vi "嵌套条件结构.vi"() -> ()   [LabVIEW 2013]
panel:
  out "output2":dbl
  out "output1":dbl
  out "?":dbl
  out "Array":bool[](array[boolean])
  in  "input":dbl
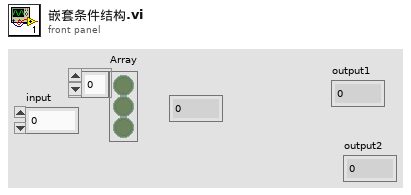
[diagram p1: front panel]
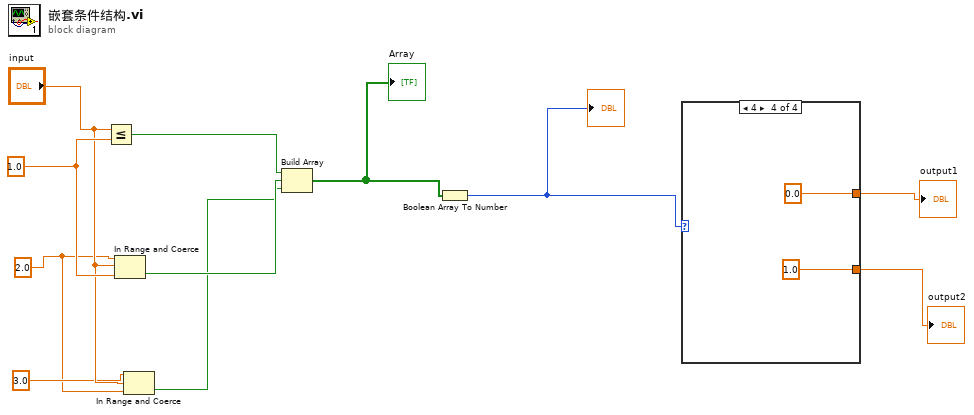
[diagram p0: block diagram]
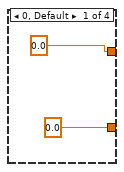
[diagram p2: hidden frame]
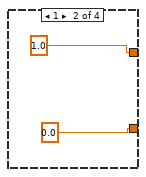
[diagram p3: hidden frame]
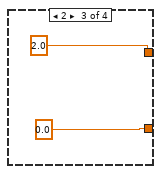
[diagram p4: hidden frame]
diagram:
  w8 = 2.0
  w11 = 1.0
  n1 = Less Or Equal?(x="input", y=w11) -> (x <= y?=w7:bool)
  n2 = In Range and Coerce(upper limit=w8, x="input", lower limit=w11) -> (In Range?=w6:bool)  [unwired: 1 out]
  n3 = In Range and Coerce(upper limit=3.0, x="input", lower limit=w8) -> (In Range?=w5:bool)  [unwired: 1 out]
  n4 = Build Array(w7, w6, w5) -> (w4:bool[])
  "Array" <- w4
  n5 = Boolean Array To Number(Boolean array=w4) -> (number=w3:u32)
  "?" <- w3
  n6 = case shown="4" w3 {
    tunnel: [0.0 1.0 2.0 0.0] -> w2
    tunnel: [0.0 0.0 0.0 1.0] -> w1
    frame 0, Default {
    }
    frame 1 {
    }
    frame 2 {
    }
    frame 4 {
    }
  }
  "output1" <- w2
  "output2" <- w1
